vi "Helper - AngleInRange.vi"(9 "Angle to check":dbl, 10 "Angle 2":dbl, 11 "Angle 1":dbl) -> (2 "In range?":bool)   [LabVIEW 2011]
doc: "Takes in wind angle + irons range and wind angle - irons range, both normalized to be within 0-360, and checks whether the angle inputed falls within the irons range."
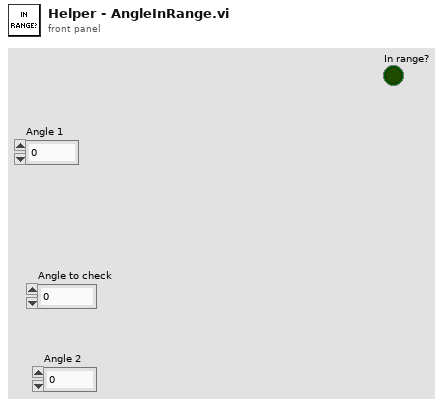
[diagram p1: front panel]
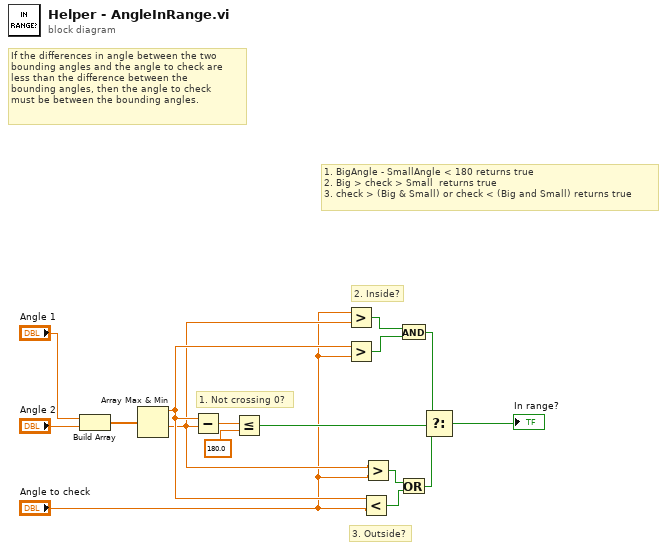
[diagram p0: block diagram]
diagram:
  # "3. Outside?"
  # "2. Inside?"
  # "1. BigAngle - SmallAngle < 180 returns true\n2. Big > check > Small  returns true\n3. check > (Big & Small) or check < (Big and Small) returns true"
  # "1. Not crossing 0?"
  # "If the differences in angle between the two\nbounding angles and the angle to check are \nless than the difference between the\nbounding angles, then the angle to check\nmust be between the bounding angles."
  n1 = Build Array("Angle 1", "Angle 2") -> (w14:dbl[])
  n2 = Array Max & Min(array=w14) -> (max value=w5:dbl, min value=w4:dbl)  [unwired: 2 out]
  n3 = Subtract(x=w5, y=w4) -> (x-y=w13:dbl)
  n4 = Less Or Equal?(x=w13, y=180.0) -> (x <= y?=w11:bool)
  n5 = Greater?(x="Angle to check", y=w4) -> (0:w10:bool)
  n6 = Greater?(x=w5, y="Angle to check") -> (0:w9:bool)
  n7 = Less?(x=w5, y="Angle to check") -> (x < y?=w1:bool)
  n8 = Greater?(x=w4, y="Angle to check") -> (0:w2:bool)
  n9 = And(x=w10, y=w9) -> (x .and. y?=w8:bool)
  n10 = Or(x=w2, y=w1) -> (x .or. y?=w7:bool)
  n11 = Select(t=w8, s=w11, f=w7) -> (s? t:f=→"In range?":bool)
